vi "SoundLevelMeasurementMarcoGonzalez.vi"() -> ()   [LabVIEW 2012]
panel:
  out "NO TALKING":bool
  out "QUIET DOWN":bool
  out "OK":bool
  out "Waveform Chart":dbl(graph)
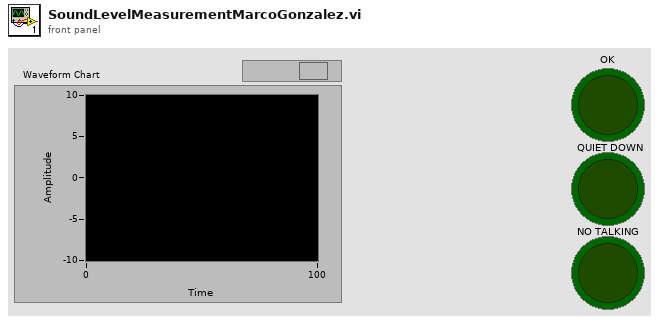
[diagram p1: front panel]
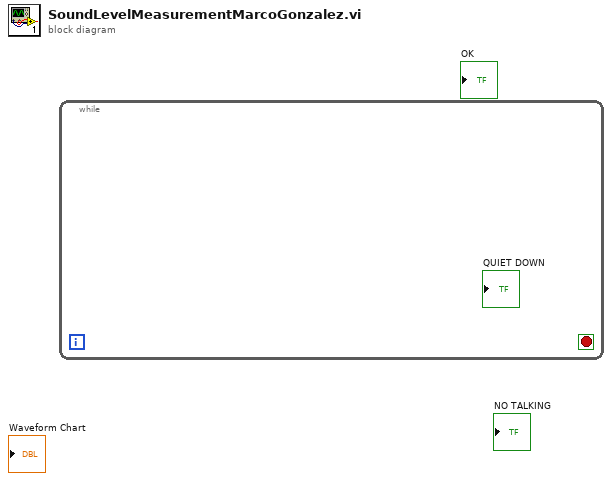
[diagram p0: block diagram]
diagram:
  n1 = while {
    stop <- _ stop-if-true
  }
